vi "BasicPID.vi"(4 "Encoder Rates":dbl[](array[numeric]), 5 "PID constants":dbl[](array[numeric]), 6 "Motor Targets":dbl[](array[numeric]), 7 "Max robot rate":dbl) -> (0 "Right Rear":dbl, 1 "Left Rear":dbl, 2 "Right Front":dbl, 3 "Left Front":dbl)   [LabVIEW 2014]
panel:
  # "Left Front"
  # "Right Front"
  # "Left Front"
  # "Left Rear"
  # "Right Front"
  # "Right Rear"
  # "Left Rear"
  # "Right Rear"
  # "Proportional"
  # "Integral"
  # "Derivative"
  # "Left Front"
  # "Right Front"
  # "Left Rear"
  # "Right Rear"
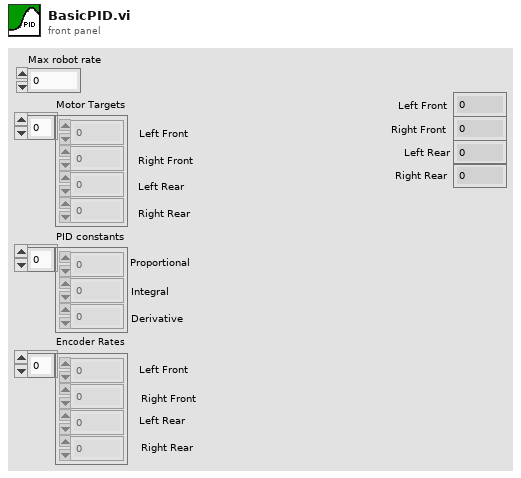
[diagram p1: front panel]
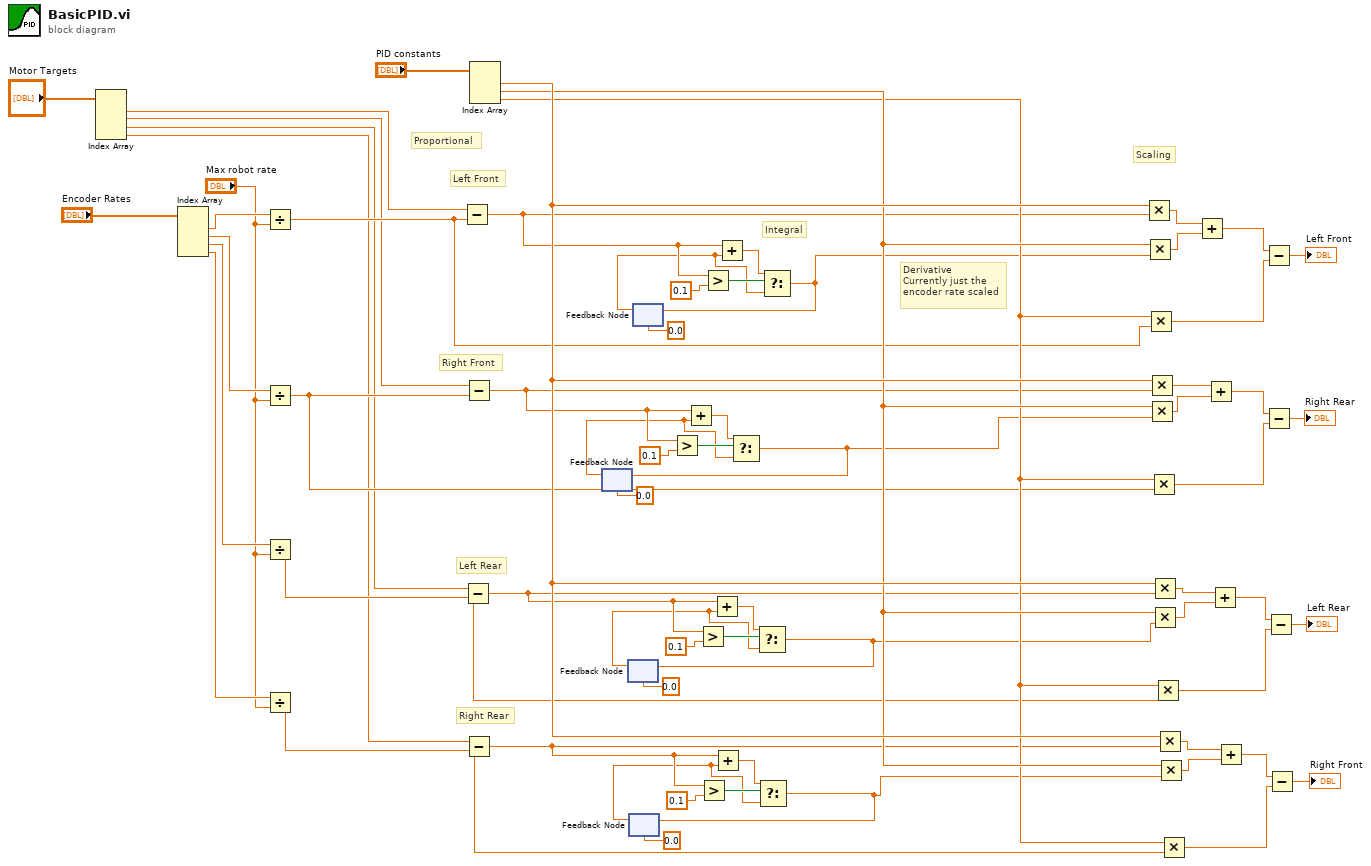
[diagram p0: block diagram]
diagram:
  # "Derivative\nCurrently just the\nencoder rate scaled"
  # "Integral"
  # "Scaling"
  # "Right Rear"
  # "Left Rear"
  # "Right Front"
  # "Left Front"
  # "Proportional"
  n1 = Index Array(array="Motor Targets") -> (element #1=w36:dbl, element #2=w35:dbl, element #3=w34:dbl, element #4=w33:dbl)  [unwired: 4 in]
  n2 = Index Array(array="Encoder Rates") -> (element #1=w32:dbl, element #2=w31:dbl, element #3=w30:dbl, element #4=w29:dbl)  [unwired: 4 in]
  n3 = Divide(x=w32, y="Max robot rate") -> (x/y=w40:dbl)
  n4 = Divide(x=w31, y="Max robot rate") -> (x/y=w39:dbl)
  n5 = Divide(x=w30, y="Max robot rate") -> (x/y=w38:dbl)
  n6 = Divide(x=w29, y="Max robot rate") -> (x/y=w37:dbl)
  n7 = Subtract(x=w36, y=w40) -> (x-y=w18:dbl)
  n8 = Subtract(x=w34, y=w38) -> (x-y=w12:dbl)
  n9 = Subtract(x=w35, y=w39) -> (x-y=w25:dbl)
  n10 = Subtract(x=w33, y=w37) -> (x-y=w6:dbl)
  n11 = Index Array(array="PID constants") -> (element #1=w65:dbl, element #2=w63:dbl, element #3=w62:dbl)  [unwired: 3 in]
  n12 = feedback #1(0.0) -> (w3:dbl)
  n13 = feedback #2(0.0) -> (w2:dbl)
  n14 = feedback #3(0.0) -> (w1:dbl)
  n15 = feedback #4(0.0) -> (w4:dbl)
  n16 = Greater?(x=w25, y=0.1) -> (0:w26:bool)
  n17 = Add(x=w25, y=w3) -> (x+y=w24:dbl)
  n18 = Greater?(x=w12, y=0.1) -> (0:w14:bool)
  n19 = Greater?(x=w6, y=0.1) -> (0:w8:bool)
  n20 = Greater?(x=w18, y=0.1) -> (0:w20:bool)
  n21 = Add(x=w12, y=w2) -> (x+y=w13:dbl)
  n22 = Add(x=w6, y=w1) -> (x+y=w7:dbl)
  n23 = Add(x=w18, y=w4) -> (x+y=w19:dbl)
  n24 = Select(t=w24, s=w26, f=w3) -> (s? t:f=w23:dbl)
  n25 = feedback-in #1(w23) -> ()
  n26 = Select(t=w13, s=w14, f=w2) -> (s? t:f=w11:dbl)
  n27 = feedback-in #2(w11) -> ()
  n28 = Select(t=w7, s=w8, f=w1) -> (s? t:f=w5:dbl)
  n29 = feedback-in #3(w5) -> ()
  n30 = Select(t=w19, s=w20, f=w4) -> (s? t:f=w17:dbl)
  n31 = feedback-in #4(w17) -> ()
  n32 = Multiply(x=w65, y=w18) -> (x*y=w59:dbl)
  n33 = Multiply(x=w63, y=w17) -> (x*y=w60:dbl)
  n34 = Multiply(x=w62, y=w40) -> (x*y=w61:dbl)
  n35 = Multiply(x=w65, y=w25) -> (x*y=w54:dbl)
  n36 = Multiply(x=w63, y=w23) -> (x*y=w55:dbl)
  n37 = Multiply(x=w62, y=w39) -> (x*y=w56:dbl)
  n38 = Multiply(x=w65, y=w12) -> (x*y=w50:dbl)
  n39 = Multiply(x=w63, y=w11) -> (x*y=w51:dbl)
  n40 = Multiply(x=w62, y=w38) -> (x*y=w52:dbl)
  n41 = Multiply(x=w65, y=w6) -> (x*y=w46:dbl)
  n42 = Multiply(x=w63, y=w5) -> (x*y=w47:dbl)
  n43 = Multiply(x=w62, y=w37) -> (x*y=w48:dbl)
  n44 = Add(x=w59, y=w60) -> (x+y=w58:dbl)
  n45 = Add(x=w54, y=w55) -> (x+y=w57:dbl)
  n46 = Add(x=w50, y=w51) -> (x+y=w53:dbl)
  n47 = Add(x=w46, y=w47) -> (x+y=w49:dbl)
  n48 = Subtract(x=w58, y=w61) -> (x-y=→"Left Front":dbl)
  n49 = Subtract(x=w57, y=w56) -> (x-y=→"Right Rear":dbl)
  n50 = Subtract(x=w53, y=w52) -> (x-y=→"Left Rear":dbl)
  n51 = Subtract(x=w49, y=w48) -> (x-y=→"Right Front":dbl)
